vi "Hysteresis Math.vi"(0 "Calibration Points in":T1[](array[typedef]), 11 "error in (no error)":errorcluster) -> (4 "Calibration Points out":T1[](array[typedef]), 6 "Current Calibration Point":T1, 8 "Next Calibration Point":T1, 10 "Hysteresis":dbl, 15 "error out":errorcluster)   [LabVIEW 2026, in "Analysis.lvlib"]
uses:
  Analysis.lvlib
  controls/Messaging Payloads/Calibration Point Table Insert.ctl
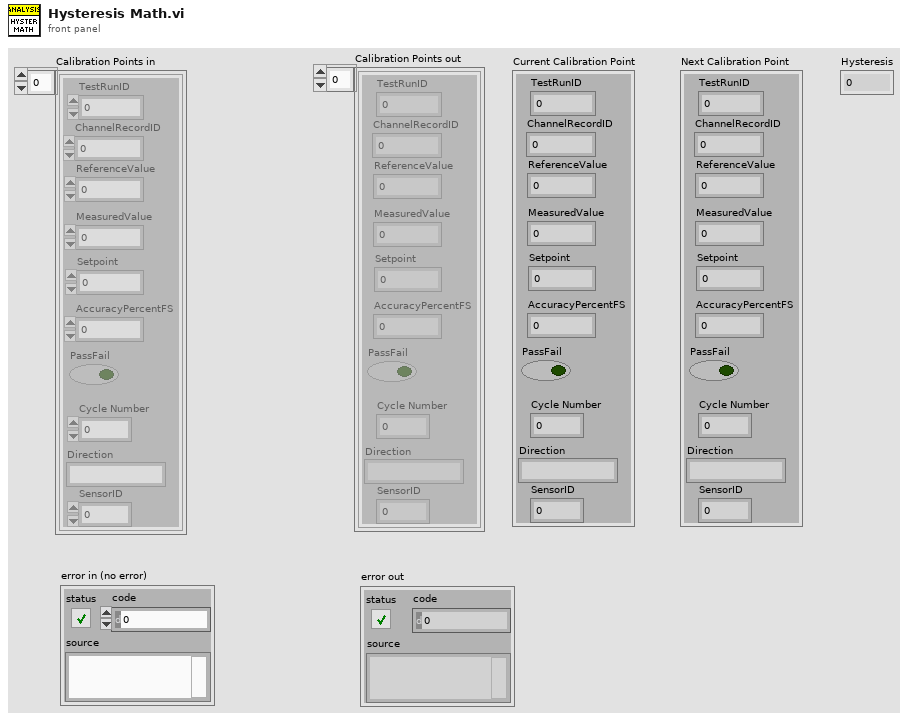
[diagram p1: front panel]
types:
  T1 = typedef "Calibration Point Table Insert.ctl" = cluster{"TestRunID":i32, "ChannelRecordID":i32, "Setpoint":dbl, "MeasuredValue":dbl, "AccuracyPercentFS":dbl, "PassFail":bool, "ReferenceValue":dbl, "Cycle Number":i32, "Direction":string, "SensorID":i32}
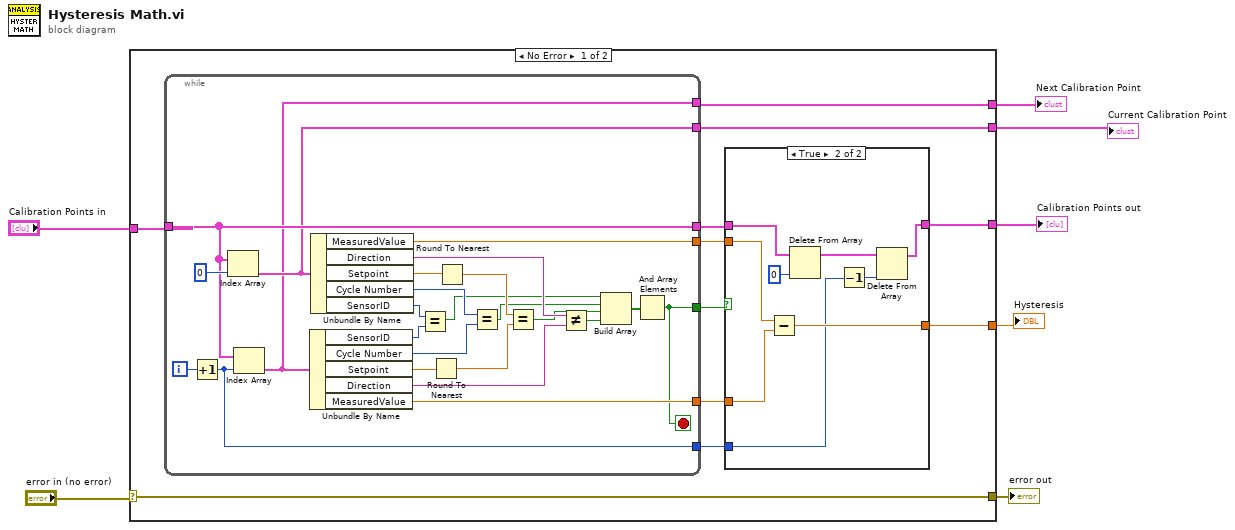
[diagram p0: block diagram]
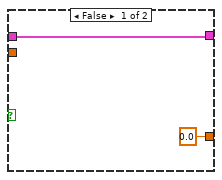
[diagram p2: hidden frame]
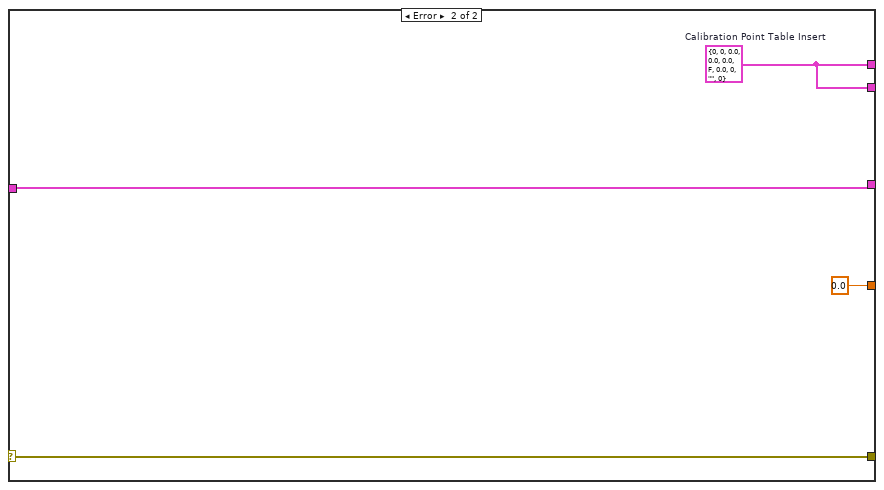
[diagram p3: hidden frame]
diagram:
  n1 = case shown="No Error" "error in (no error)" {
    selector: "error in (no error)" -> [w8 w56]
    tunnel: [w18 0.0] -> w7
    tunnel: [w17 w54] -> w6
    tunnel: [w16 w54] -> w5
    tunnel: "Calibration Points in" -> [w14 w57]
    tunnel: [w9 w57] -> w3
    tunnel: [w8 w56] -> w1
    frame No Error {
      n2 = while {
        tunnel: w14 -> [w23]
        tunnel: [w24] -> w10
        tunnel: [w26] -> w11
        tunnel: [w25] -> w12
        tunnel: [w23] -> w13
        tunnel: [w21] -> w15
        tunnel: [w20] -> w16
        tunnel: [w19] -> w17
        i -> [w22]
        stop <- w24 stop-if-true
        n3 = Increment(x=w22) -> (x+1=w21:i32)
        n4 = Index Array(array=w23, index=0) -> (element=w20:T1)
        n5 = Index Array(array=w23, index=w21) -> (element=w19:T1)
        n6 = Unbundle By Name(w19) -> ("SensorID"=w40:i32, "Cycle Number"=w38:i32, "Setpoint"=w35:dbl, "Direction"=w32:string, "MeasuredValue"=w25:dbl)
        n7 = Unbundle By Name(w20) -> ("MeasuredValue"=w26:dbl, "Direction"=w33:string, "Setpoint"=w37:dbl, "Cycle Number"=w39:i32, "SensorID"=w41:i32)
        n8 = Equal?(x=w41, y=w40) -> (x = y?=w28:bool)
        n9 = Round To Nearest(number=w35) -> (nearest integer value=w34:dbl)
        n10 = Round To Nearest(number=w37) -> (nearest integer value=w36:dbl)
        n11 = Equal?(x=w39, y=w38) -> (x = y?=w29:bool)
        n12 = Equal?(x=w36, y=w34) -> (x = y?=w30:bool)
        n13 = Not Equal?(x=w33, y=w32) -> (x != y?=w31:bool)
        n14 = Build Array(w28, w29, w30, w31) -> (w27:bool[])
        n15 = And Array Elements(Boolean array=w27) -> (logical AND=w24:bool)
      }
      n16 = case shown="True" w10 {
        tunnel: [w44 w47] -> w9
        tunnel: w13 -> [w44 w53]
        tunnel: w11 -> [_ w50]
        tunnel: w12 -> [_ w51]
        tunnel: [0.0 w49] -> w18
        tunnel: w15 -> [_ w46]
        frame False {
        }
        frame True {
          n17 = Subtract(x=w50, y=w51) -> (x-y=w49:dbl)
          n18 = Delete From Array(array=w53, index=0) -> (array with subset deleted=w48:T1[])  [unwired: 1 in, 1 out]
          n19 = Decrement(x=w46) -> (x-1=w45:i32)
          n20 = Delete From Array(array=w48, index=w45) -> (array with subset deleted=w47:T1[])  [unwired: 1 in, 1 out]
        }
      }
    }
    frame Error {
      w54 = T1 {"TestRunID"=0, "ChannelRecordID"=0, "Setpoint"=0.0, "MeasuredValue"=0.0, "AccuracyPercentFS"=0.0, "PassFail"=FALSE, "ReferenceValue"=0.0, "Cycle Number"=0, "Direction"="", "SensorID"=0}  # Calibration Point Table Insert
    }
  }
  "Hysteresis" <- w7
  "Next Calibration Point" <- w6
  "Current Calibration Point" <- w5
  "Calibration Points out" <- w3
  "error out" <- w1
